vi "Read proto.vi"(10 "String":string="syntax = \"proto2\";\n\nmessage Feedback {\nrequired uint32 id = 1;\nrequired uint32 status = 2;\nrequired float battery = 3;\nrequired float encoder1 = 4;\nrequired float encoder2 = 5;\nrequired float encoder3 = 6;\nrequired float encoder4 = 7;\n}") -> (1 "syntax":string, 2 "Cluster Array":T1(array[cluster]), 3 "message":string)   [LabVIEW 2020]
uses:
  <vilib>/Utility/error.llb/whitespace.ctl
panel:
  out "remaining string":string
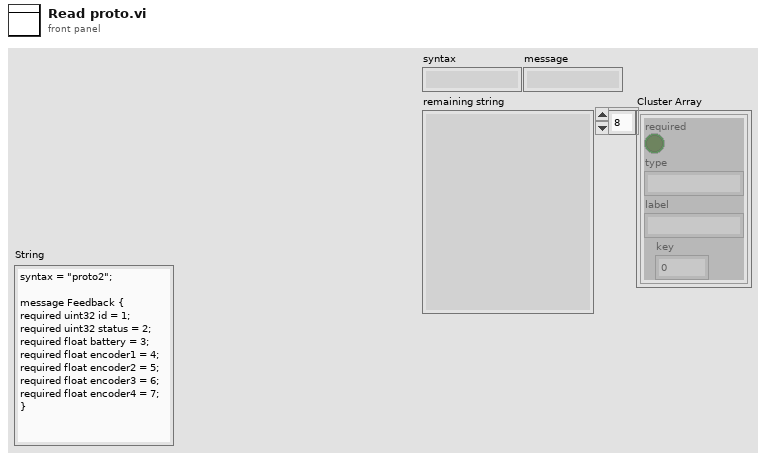
[diagram p1: front panel]
types:
  T1 = cluster{"required":bool, "type":string, "label":string, "key":i32}[]
  T2 = cluster{"required":bool, "type":string, "label":string, "key":i32}
  T3 = typedef "whitespace.ctl" = u16
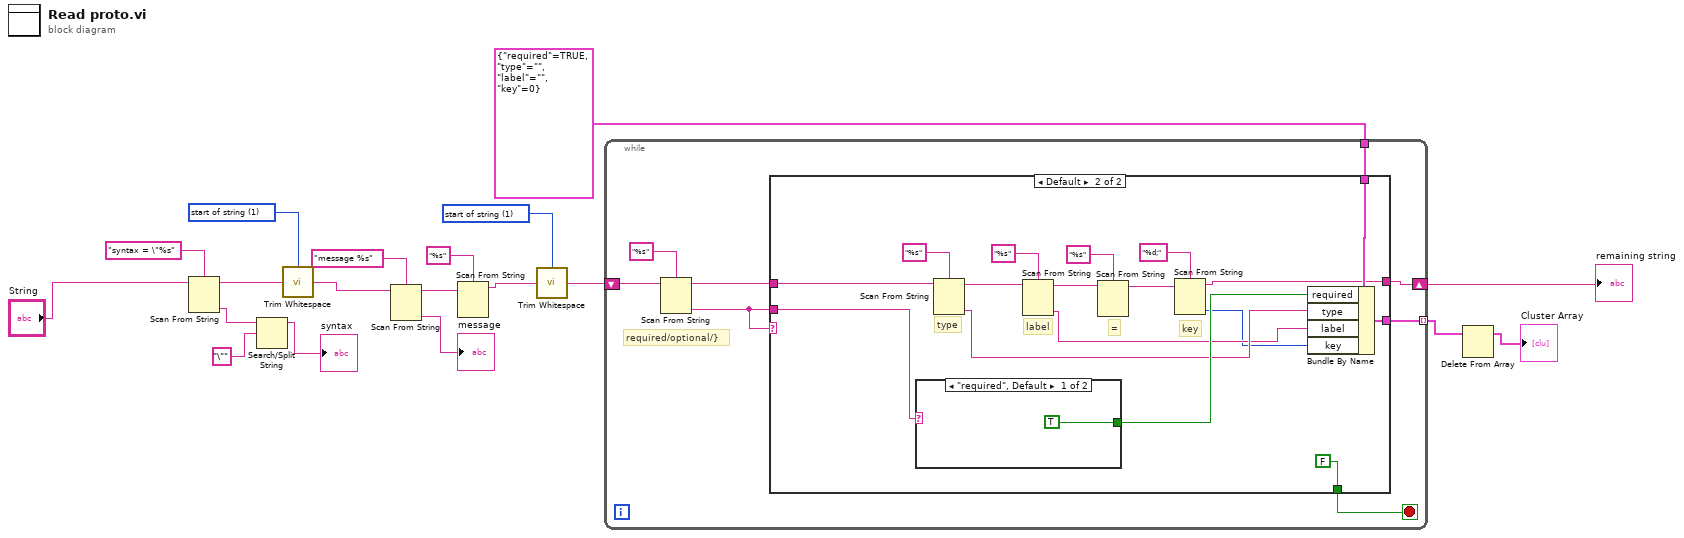
[diagram p0: block diagram]
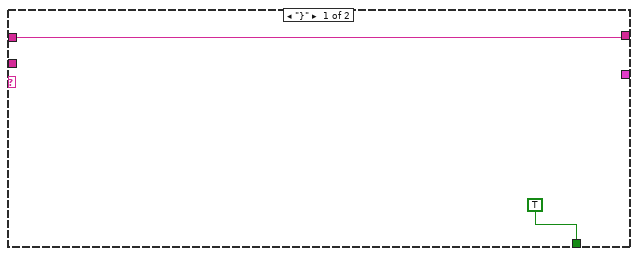
[diagram p2: hidden frame]
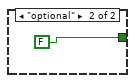
[diagram p3: hidden frame]
diagram:
  w7 = T3 1 items=["both", "start of string", "end of string"] ("location (both)")
  w12 = T3 1 items=["both", "start of string", "end of string"] ("location (both)")
  n1 = Scan From String(format string="syntax = \"%s", input string="String") -> (remaining string=w11:string, output 1=w17:string)  [unwired: 3 in, 2 out]
  n2 = Search/Split String(string=w17, search string/char (-)="\"") -> (substring before match=→"syntax":string)  [unwired: 1 in, 2 out]
  n3 = call <vilib>:"Trim Whitespace.vi"("string"=w11, "location (both)"=w12) -> ("trimmed string"=w10:string)
  n4 = Scan From String(format string="message %s", input string=w10) -> (remaining string=w9:string, output 1=→"message":string)  [unwired: 3 in, 2 out]
  n5 = Scan From String(format string="%s", input string=w9) -> (remaining string=w6:string)  [unwired: 4 in, 2 out]
  n6 = call <vilib>:"Trim Whitespace.vi"("string"=w6, "location (both)"=w7) -> ("trimmed string"=w5:string)
  n7 = while {
    tunnel: T2 {"required"=TRUE, "type"="", "label"="", "key"=0} -> [w24]
    tunnel: [w23] -> w2 mode=indexing
    shift-right: [w22] -> w3
    shift-left: w5 -> [w27]
    stop <- w20 stop-if-true
    # "required/optional/}"
    n8 = Scan From String(format string="%s", input string=w27) -> (remaining string=w25:string, output 1=w21:string)  [unwired: 3 in, 2 out]
    n9 = case shown="Default" w21 {
      tunnel: w25 -> [w29 w46]
      tunnel: w24 -> [_ w40]
      tunnel: w21 -> [_ w39]
      tunnel: [_ w34] -> w23
      tunnel: [w29 w31] -> w22
      tunnel: [TRUE FALSE] -> w20
      frame "}" {
      }
      frame Default {
        # "key"
        # "="
        # "label"
        # "type"
        n10 = case shown="\"required\", Default" w39 {
          tunnel: [TRUE FALSE] -> w38
          frame "required", Default {
          }
          frame "optional" {
          }
        }
        n11 = Scan From String(format string="%s", input string=w46) -> (remaining string=w44:string, output 1=w37:string)  [unwired: 3 in, 2 out]
        n12 = Scan From String(format string="%s", input string=w44) -> (remaining string=w33:string, output 1=w36:string)  [unwired: 3 in, 2 out]
        n13 = Scan From String(format string="%s", input string=w33) -> (remaining string=w32:string)  [unwired: 4 in, 2 out]
        n14 = Scan From String(format string="%d;", input string=w32) -> (remaining string=w31:string, output 1=w35:i32)  [unwired: 3 in, 2 out]
        n15 = Bundle By Name(cluster=w40, "required"=w38, "type"=w37, "label"=w36, "key"=w35) -> (w34:T2)
      }
    }
  }
  "remaining string" <- w3
  n16 = Delete From Array(array=w2) -> (array with subset deleted=→"Cluster Array":T1)  [unwired: 2 in, 1 out]
